vi "Lab 1 Set Freq.vi"() -> ()   [LabVIEW 2015]
uses:
  <instrlib>/Siglent SDG 1000 5000 800 Series/Siglent SDG 1000 5000 800 Series.lvlib
panel:
  in  "Frequency (1000 Hz)":dbl=1000.0 min=1e-06 max=160000000.0 step=1.0 format="%#.6g"
  out "error out":errorcluster
  out "VISA resource name out":refnum<visa-resource-name>
  in  "?":errorcluster
  in  "VISA resource name":refnum<visa-resource-name>
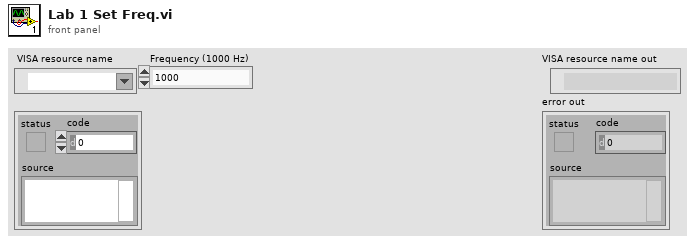
[diagram p1: front panel]
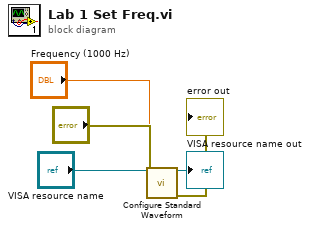
[diagram p0: block diagram]
diagram:
  n1 = call <instrlib>:"Configure Standard Waveform.vi"("VISA resource name"="VISA resource name", "Frequency (1000 Hz)"="Frequency (1000 Hz)", "error in (no error)"="?") -> ("VISA resource name out"=→"VISA resource name out":refnum<visa-resource-name>, "error out"=→"error out":errorcluster)  [unwired: 11 in]
